vi "Complex Double.vi"(7 "data type of variable":cdb, 8 "error in":errorcluster, 10 "variable name":string, 11 "pipe in":T1) -> (0 "error out":errorcluster, 2 "value":cdb format="%.2f", 3 "pipe out":T1)   [LabVIEW 2013, in "GOLPI library.lvlib"]
uses:
  GOLPI library.lvlib
  LV Process.lvlibp/Pipe Handle.ctl
  Globals.vi
  <vilib>/Utility/error.llb/Error Cluster From Error Code.vi
  <vilib>/regexp/Match Regular Expression.xnode
  <vilib>/ErrorRing/Error Ring.xnode
  LV Process.lvlibp
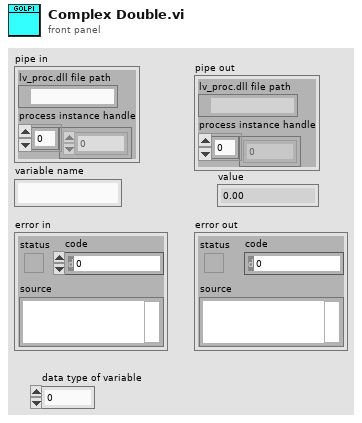
[diagram p1: front panel]
types:
  T1 = typedef "LV Process.lvlibp/Pipe Handle.ctl" = cluster{"lv_proc.dll file path":path, "process instance handle":u32[]}
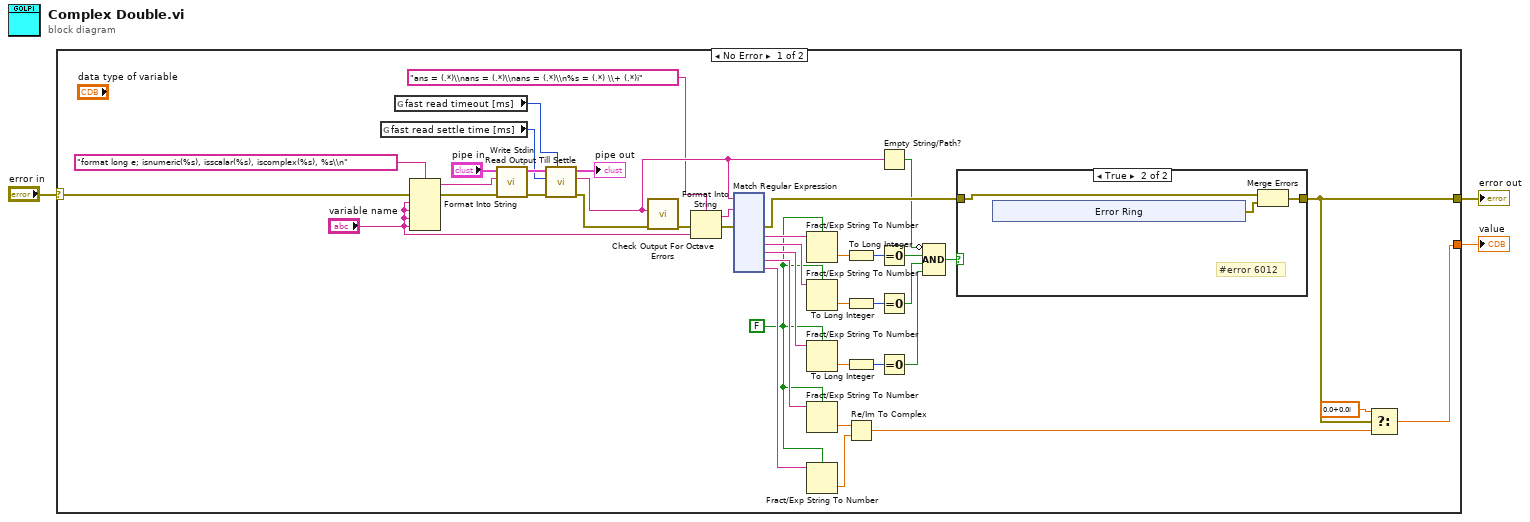
[diagram p0: block diagram]
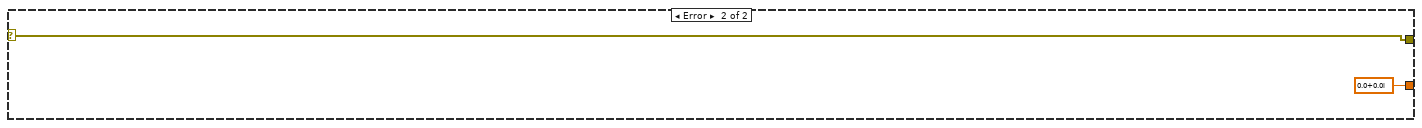
[diagram p3: hidden frame]
diagram:
  n1 = case shown="No Error" "error in" {
    selector: "error in" -> [w15 w175]
    tunnel: [w19 cdb 0.0+0.0i ("t")] -> w3
    tunnel: [w18 w175] -> w2
    frame No Error {
      w7 = FALSE ("use system decimal point (T)")
      n2 = global read "Globals.vi" "fast read settle time [ms]"() -> (w26:u32)
      n3 = global read "Globals.vi" "fast read timeout [ms]"() -> (w25:u32)
      n4 = Format Into String(format string="format long e; isnumeric(%s), isscalar(%s), iscomplex(%s), %s\\n", error in=w15, "variable name", "variable name", "variable name", "variable name") -> (resulting string=w37:string, error out=w14:errorcluster)  [unwired: 1 in]
      n5 = call "Write Stdin.vi"("error in"=w14, "write buffer"=w37, "pipe in"="pipe in") -> ("error out"=w27:errorcluster, "pipe out"=w43:T1)  [unwired: 6 in, 1 out]
      n6 = call "Read Output Till Settle.vi"("timeout [ms]"=w25, "error in"=w27, "settled for [ms]"=w26, "pipe in"=w43) -> ("error out"=w29:errorcluster, "read buffer"=w17:string, "pipe out"=→"pipe out":T1)  [unwired: 4 in, 1 out]
      n7 = call "Check Output For Octave Errors.vi"("error in"=w29, "read buffer"=w17) -> ("error out"=w11:errorcluster)  [unwired: 9 in]
      n8 = Format Into String(format string="ans = (.*)\\nans = (.*)\\nans = (.*)\\n%s = (.*) \\+ (.*)i" ("regular expression"), error in=w11, "variable name") -> (resulting string=w12:string, error out=w10:errorcluster)  [unwired: 1 in]
      n9 = xnode "Match Regular Expression"("input string"=w17, "regular expression"=w12, "error in"=w10) -> ("error out"=w28:errorcluster, "submatch 1"=w41:string, "submatch 2"=w36:string, "submatch 3"=w35:string, "submatch 4"=w34:string, "submatch 5"=w8:string)  [unwired: 3 in, 4 out]
      n10 = Fract/Exp String To Number(use system decimal point (T)=w7, string=w41) -> (number=w40:dbl)  [unwired: 2 in, 1 out]
      n11 = Fract/Exp String To Number(use system decimal point (T)=w7, string=w36) -> (number=w32:dbl)  [unwired: 2 in, 1 out]
      n12 = Fract/Exp String To Number(use system decimal point (T)=w7, string=w35) -> (number=w33:dbl)  [unwired: 2 in, 1 out]
      n13 = Fract/Exp String To Number(use system decimal point (T)=w7, string=w34) -> (number=w5:dbl)  [unwired: 2 in, 1 out]
      n14 = Fract/Exp String To Number(use system decimal point (T)=w7, string=w8) -> (number=w6:dbl)  [unwired: 2 in, 1 out]
      n15 = To Long Integer(number=w40) -> (32bit integer=w39:i32)
      n16 = To Long Integer(number=w32) -> (32bit integer=w31:i32)
      n17 = To Long Integer(number=w33) -> (32bit integer=w30:i32)
      n18 = Re/Im To Complex(1:w6, 2:w5) -> (0:w4:cdb)
      n19 = Empty String/Path?(string/path=w17) -> (empty?=w21:bool)
      n20 = Equal To 0?(x=w39) -> (x = 0?=w24:bool)
      n21 = Equal To 0?(x=w31) -> (x = 0?=w23:bool)
      n22 = Equal To 0?(x=w30) -> (x = 0?=w22:bool)
      n23 = Compound Arithmetic op=AND(invert w21, w24, w23, w22) -> (w20:bool)
      n24 = case shown="True" w20 {
        tunnel: [w45 w46] -> w18
        tunnel: w28 -> [w45 w47]
        frame False {
        }
        frame True {
          # "#error 6012"
          n25 = xnode "Error Ring"() -> ("error out"=w48:errorcluster)
          n26 = Merge Errors(w47, w48) -> (w46:errorcluster)
        }
      }
      n27 = Select(t=cdb 0.0+0.0i, s=w18, f=w4) -> (s? t:f=w19:cdb)
    }
    frame Error {
    }
  }
  "value" <- w3
  "error out" <- w2
